vi "Query S Parameters.vi"(8 "error in (no error)":errorcluster, 10 "Sparameters (string)":string[](array[string]), 11 "VNA-ENA in":refnum<class "VNA-ENA.lvclass">) -> (0 "error out":errorcluster, 2 "S parameters":T1[](array[typedef]), 3 "VNA-ENA out":refnum<class "VNA-ENA.lvclass">)   [LabVIEW 2020, in "VNA-ENA.lvclass"]
doc: "Queryes the S parameter choosen. It can give single parameter or full 2 to 4 port parameters.\nFor one port S Parameter array only have Sxx.\nFor N ports the S Parameter array hold S11,S12,...,S1N,S21,S22,...,SNN"
uses:
  VNA-ENA.lvclass
  C:/Sandbox/RF Bench/Source Code/WiSpry Test Framework/Instruments/Instrument.lvclass
  Controls/Sparameter cluster.ctl
  Instrument.lvclass/Instrument.ctl
  Instrument.lvclass
  Vector Network Analyzer.lvclass
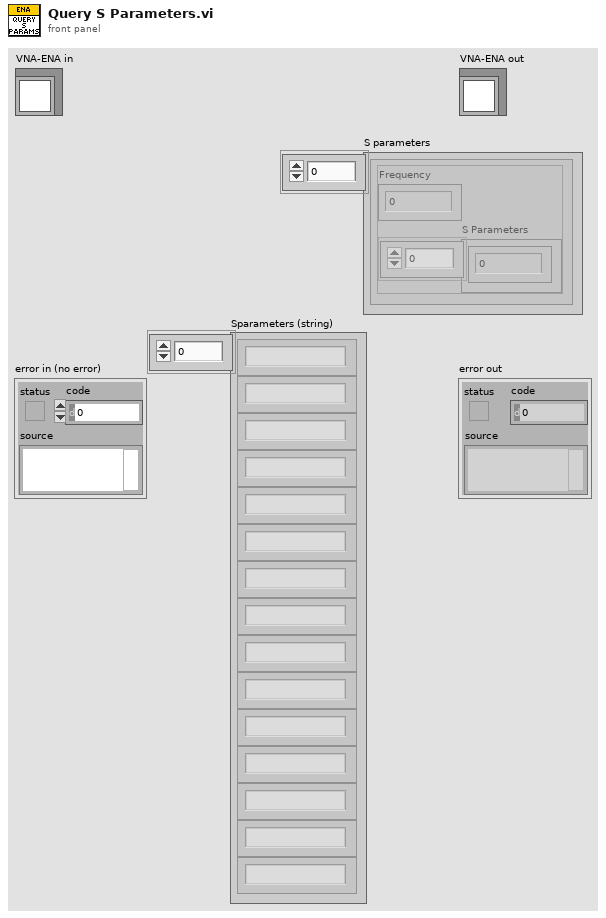
[diagram p1: front panel]
types:
  T1 = typedef "Vector Network Analyzer.lvclass/Sparameter cluster.ctl" = cluster{"Frequency":dbl, "S Parameters":cdb[]}
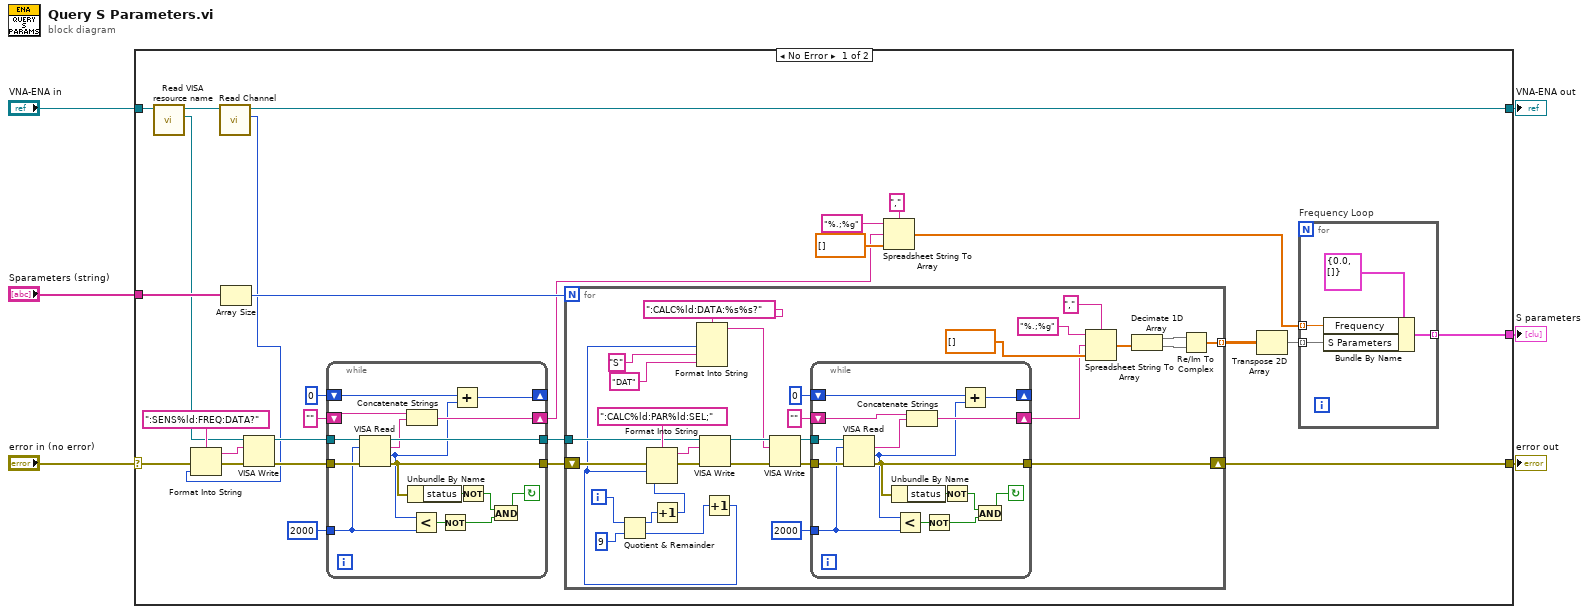
[diagram p0: block diagram]
diagram:
  n1 = case shown="No Error" "error in (no error)" {
    selector: "error in (no error)" -> [w16 w101]
    tunnel: [w29 w101] -> w5
    tunnel: [w26 w100] -> w4
    tunnel: "VNA-ENA in" -> [w33 w100]
    tunnel: "Sparameters (string)" -> [w32 _]
    tunnel: [w30 _] -> w1
    frame No Error {
      n2 = call "Read VISA resource name.vi"("Instrument in"=w33) -> ("VISA resource name"=w19:refnum<visa-resource-name>, "Instrument out"=w25:refnum<class "VNA-ENA.lvclass">)  [unwired: 9 in]
      n3 = call-dynamic "Read Channel.vi"("Vector Network Analyzer in"=w25) -> ("Channel"=w7:i32, "Vector Network Analyzer out"=w26:refnum<class "VNA-ENA.lvclass">)  [unwired: 9 in]
      n4 = Format Into String(format string=":SENS%ld:FREQ:DATA?", error in=w16, w7) -> (resulting string=w20:string, error out=w17:errorcluster)  [unwired: 1 in]
      n5 = Array Size(array=w32) -> (size(s)=w31:i32)
      n6 = VISA Write(VISA resource name=w19, write buffer=w20, error in (no error)=w17) -> (VISA resource name out=w13:refnum<visa-resource-name>, error out=w14:errorcluster)  [unwired: 1 out]
      n7 = while {
        shift-left: "" -> [w43]
        shift-right: [w44] -> w10
        tunnel: u32 2000 ("Buffer Size") -> [w34]
        shift-left: u32 0 -> [w47]
        shift-right: [w46] -> _
        tunnel: [w48] -> w12
        tunnel: w13 -> [w49]
        tunnel: w14 -> [w40]
        tunnel: [w41] -> w11
        stop <- w36 continue-if-true
        n8 = VISA Read(VISA resource name=w49, byte count=w34, error in (no error)=w40) -> (VISA resource name out=w48:refnum<visa-resource-name>, read buffer=w42:string, return count=w35:u32, error out=w41:errorcluster)
        n9 = Concatenate Strings(w43, w42) -> (w44:string)
        n10 = Unbundle By Name(w41) -> ("status"=w45:bool)
        n11 = Less?(x=w35, y=w34) -> (x < y?=w39:bool)
        n12 = Not(x=w39) -> (.not. x?=w38:bool)
        n13 = Add(x=w47, y=w35) -> (x+y=w46:u32)
        n14 = Not(x=w45) -> (.not. x?=w37:bool)
        n15 = And(x=w37, y=w38) -> (x .and. y?=w36:bool)
      }
      n16 = for {
        N: w31 -> [_]
        tunnel: w12 -> [w75]
        tunnel: [w80] -> w28 mode=indexing
        shift-right: [w64] -> w29
        shift-left: w11 -> [w76]
        i -> [w58]
        n17 = Quotient & Remainder(x=w58, y=9) -> (x-y*floor(x/y)=w56:i32, floor(x/y)=w57:i32)
        n18 = Increment(x=w56) -> (x+1=w55:i32)
        n19 = Increment(x=w57) -> (x+1=w50:i32)
        n20 = Format Into String(format string=":CALC%ld:PAR%ld:SEL;", error in=w76, w50, w55) -> (resulting string=w78:string, error out=w79:errorcluster)  [unwired: 1 in]
        n21 = Format Into String(format string=":CALC%ld:DATA:%s%s?", w50, "S", "DAT") -> (resulting string=w51:string)  [unwired: 2 in, 1 out]
        n22 = VISA Write(VISA resource name=w75, write buffer=w78, error in (no error)=w79) -> (VISA resource name out=w68:refnum<visa-resource-name>, error out=w67:errorcluster)  [unwired: 1 out]
        n23 = VISA Write(VISA resource name=w68, write buffer=w51, error in (no error)=w67) -> (VISA resource name out=w65:refnum<visa-resource-name>, error out=w66:errorcluster)  [unwired: 1 out]
        n24 = while {
          shift-left: "" -> [w90]
          shift-right: [w91] -> w63
          tunnel: u32 2000 ("Buffer Size") -> [w81]
          shift-left: u32 0 -> [w94]
          shift-right: [w93] -> _
          tunnel: w65 -> [w95]
          tunnel: w66 -> [w87]
          tunnel: [w88] -> w64
          stop <- w83 continue-if-true
          n25 = VISA Read(VISA resource name=w95, byte count=w81, error in (no error)=w87) -> (read buffer=w89:string, return count=w82:u32, error out=w88:errorcluster)  [unwired: 1 out]
          n26 = Unbundle By Name(w88) -> ("status"=w92:bool)
          n27 = Less?(x=w82, y=w81) -> (x < y?=w86:bool)
          n28 = Concatenate Strings(w90, w89) -> (w91:string)
          n29 = Not(x=w86) -> (.not. x?=w85:bool)
          n30 = Not(x=w92) -> (.not. x?=w84:bool)
          n31 = Add(x=w94, y=w82) -> (x+y=w93:u32)
          n32 = And(x=w84, y=w85) -> (x .and. y?=w83:bool)
        }
        n33 = Spreadsheet String To Array(delimiter (Tab)=",", format string="%.;%g", spreadsheet string=w63, array type (2D Dbl)=dbl[] []) -> (array=w74:dbl[])
        n34 = Decimate 1D Array(w74) -> (w70:dbl[], w69:dbl[])
        n35 = Re/Im To Complex(1:w69, 2:w70) -> (0:w80:cdb[])
      }
      n36 = Spreadsheet String To Array(delimiter (Tab)=",", format string="%.;%g", spreadsheet string=w10, array type (2D Dbl)=dbl[] []) -> (array=w18:dbl[])
      n37 = Transpose 2D Array(2D array=w28) -> (transposed array=w27:cdb[][])
      n38 = for "Frequency Loop" {
        tunnel: [w98] -> w30 mode=indexing
        tunnel: w18 -> [w97] mode=indexing
        tunnel: w27 -> [w96] mode=indexing
        n39 = Bundle By Name(cluster=T1 {"Frequency"=0.0, "S Parameters"=[]} ("S Parameters"), "Frequency"=w97, "S Parameters"=w96) -> (w98:T1)
      }
    }
    frame Error {
    }
  }
  "error out" <- w5
  "VNA-ENA out" <- w4
  "S parameters" <- w1
